vi "Steering Controller.vi"(0 "Outer Loop State in":T1 {"Phi Setpoint" format="%#_13g"}, 7 "Steering On/off":bool, 9 "Inner Loop State in":T2, 11 "error in":errorcluster, 12 "PID Gains in":T3) -> (10 "Inner Loop State out":T2, 15 "error out":errorcluster)   [LabVIEW 2014]
uses:
  <vilib>/addons/control/pid/pid.llb/PID Structure.ctl
  <vilib>/addons/control/pid/pid.llb/PID Structure Conversion (DBL).vi
  <vilib>/addons/control/pid/pid.llb/PID (DBL).vi
  <vilib>/addons/control/pid/NI_PID_pid.lvlib
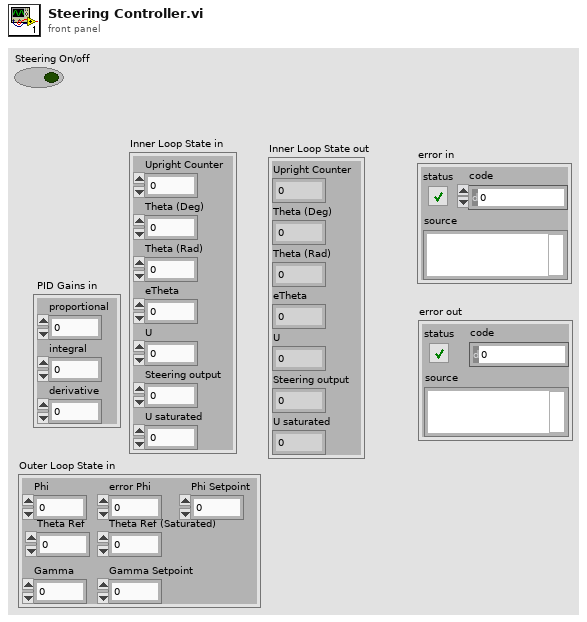
[diagram p1: front panel]
types:
  T1 = cluster{"Phi":dbl, "error Phi":dbl, "Gamma":dbl, "Theta Ref":dbl, "Theta Ref (Saturated)":sgl, "Gamma Setpoint":dbl, "Phi Setpoint":dbl}
  T2 = cluster{"Upright Counter":dbl, "Theta (Deg)":dbl, "Theta (Rad)":dbl, "eTheta":dbl, "U":dbl, "Steering output":dbl, "U saturated":sgl}
  T3 = cluster{"proportional":dbl, "integral":dbl, "derivative":dbl}
  T4 = typedef "NI_PID_pid.lvlib/PID Structure.ctl" = u16
  T5 = cluster{"proportional gain (Kc)":dbl, "integral time (Ti, min)":dbl, "derivative time (Td, min)":dbl}
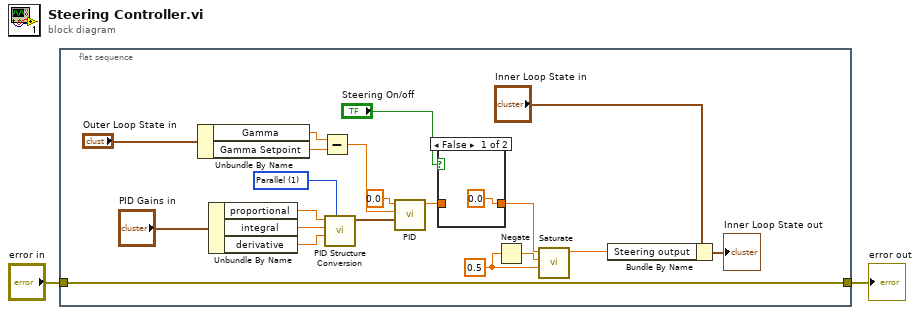
[diagram p0: block diagram]
diagram:
  n1 = flat-sequence {
    tunnel: "error in" -> [w3]
    tunnel: [w3] -> w1
    frame #0 {
      w22 = T4 1 items=["Academic (Standard)", "Parallel", "Series"] ("PID structure")
      w5 = sgl 0.5 ("min")
      n2 = Unbundle By Name("Outer Loop State in") -> ("Gamma"=w13:dbl, "Gamma Setpoint"=w8:dbl)
      n3 = Unbundle By Name("PID Gains in") -> ("proportional"=w19:dbl, "integral"=w18:dbl, "derivative"=w17:dbl)
      n4 = Subtract(x=w13, y=w8) -> (x-y=w16:dbl)
      n5 = call-poly <vilib>:"PID Structure Conversion.vi"("PID structure"=w22, "derivative"=w17, "integral"=w18, "proportional"=w19) -> ("PID gains"=w21:T5)  [unwired: 7 in]
      n6 = call-poly <vilib>:"PID.vi"("PID gains"=w21, "process variable"=w16, "setpoint"=0.0) -> ("output"=w12:dbl)  [unwired: 7 in, 1 out]
      n7 = case shown="False" "Steering On/off" {
        tunnel: w12 -> [_ w24]
        tunnel: [0.0 ("output") w24] -> w7
        frame False {
        }
        frame True {
        }
      }
      n8 = Negate(x=w5) -> (-x=w6:sgl)
      n9 = call "Saturate.vi"("Max"=w5, "Min"=w6, "X in"=w7) -> ("X out"=w4:dbl)  [unwired: 8 in]
      n10 = Bundle By Name(cluster="Inner Loop State in", "Steering output"=w4) -> (→"Inner Loop State out":T2)
    }
  }
  "error out" <- w1
